vi "Limelight Set Camera Mode.vi"(11 "Camera and Stream Mode":bool) -> ()   [LabVIEW 2020]
uses:
  <vilib>/Rock Robotics/Network Tables/NT Write Number.vi
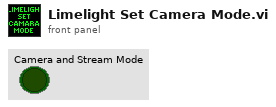
[diagram p1: front panel]
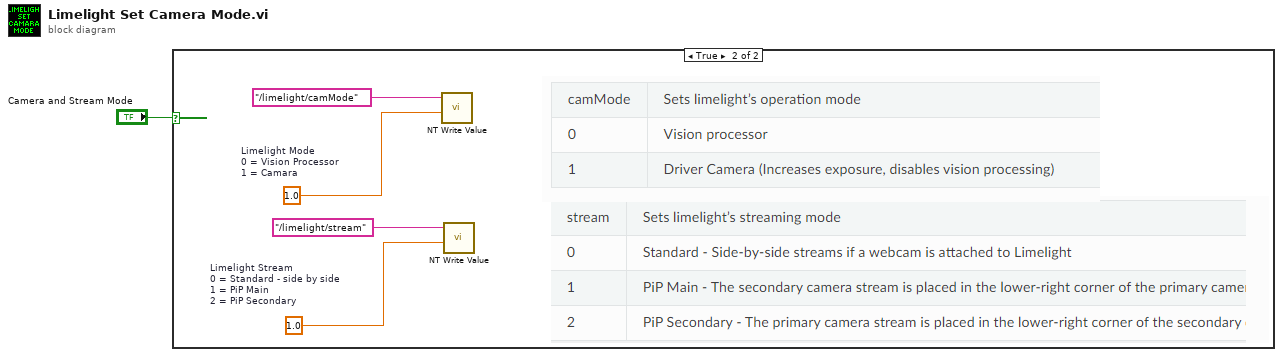
[diagram p0: block diagram]
diagram:
  n1 = case shown="True" "Camera and Stream Mode" {
    frame False {
    }
    frame True {
      w3 = 1.0  # Limelight Stream 0 = Standard - side by side 1 = PiP Main 2 = PiP Secondary
      w4 = 1.0  # Limelight Mode 0 = Vision Processor 1 = Camara
      n2 = call-poly <vilib>:"NT Write Value.vi"("Numeric"=w4, "Name"="/limelight/camMode") -> ()  [unwired: 9 in, 1 out]
      n3 = call-poly <vilib>:"NT Write Value.vi"("Numeric"=w3, "Name"="/limelight/stream") -> ()  [unwired: 9 in, 1 out]
    }
  }
